vi "Main.vi"() -> ()   [LabVIEW 2017]
uses:
  Control/Virtual Damping.ctl
  88f77483-e56a-468f-9be9-12bd898d8bad.vi
  SubVI/Global.vi
panel:
  in  "beta":dbl=0.1
  in  "Survival Rate":dbl=0.5
  in  "min(Virtual Damping)":dbl=0.5
  in  "max(Virtual Damping)":dbl=3.5
  out "Fitness Value":dbl[](array[numeric])=[0.120637, 0.055035]
  out "Population":dbl[](array[numeric])=[2.8446050566710155, 2.844440959853998, 2.8444573695357, 2.844440959853998, 2.8445886469893136, 2.8446050566710155, 2.844605056671015, 2.860850641555683]
  out "Generation":i32=6
  in  "Trials per Gen.":i32=8 min=1
  out "Trial":i32=43
  in  "Trial Time (s)":dbl=10.0 format="%#_13g"
  out "Virtual Damping":T1={"bR"=4503599627370496.0, "bP"=2.8444573695357, "bY"=4503599627370496.0}
  in  "string":string="C:\\Users\\AWEAR\\Documents\\Blender"
  in  "Epsilon (deg)":dbl=2.5
  in  "Motion (deg)":dbl=75.0 format="%#_13g"
  in  "Type":enum16{"Mini45", "Joystick", "Simulation"}(ring)=enum."Joystick"
  out "error out":errorcluster
  in  "Stop":bool
  in  "error in":errorcluster
  in  "Exit":bool
  in  "Start":bool
  in  "ADL":u16(ring)=2 items=["None", "Book", "Pitcher", "Laptop", "Gear"]
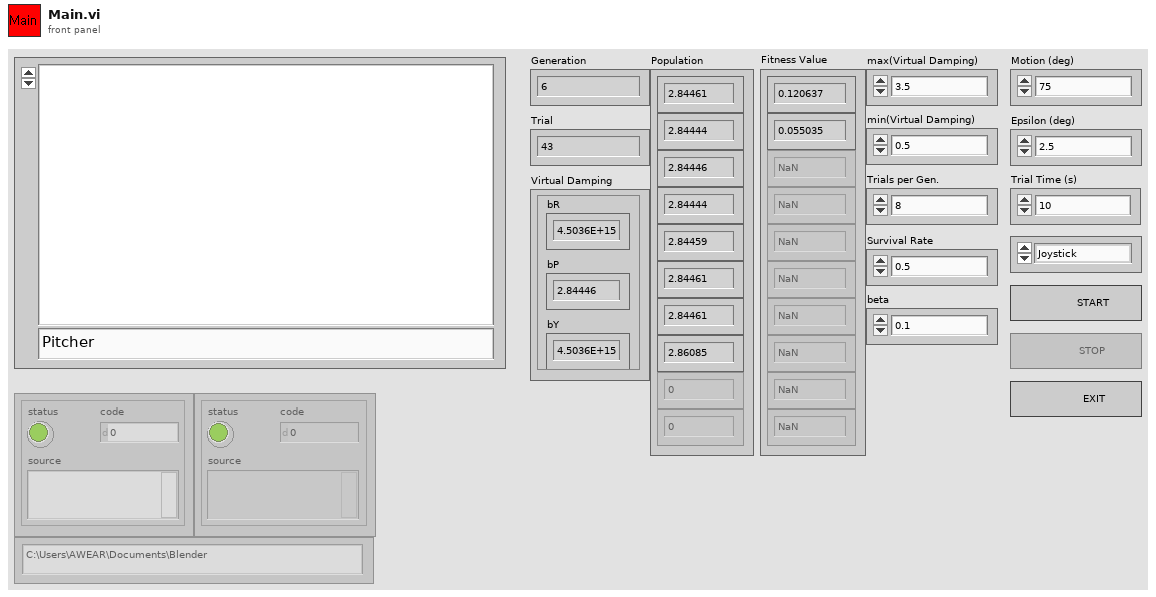
[diagram p1: front panel]
types:
  T1 = typedef "Virtual Damping.ctl" = cluster{"bR":dbl, "bP":dbl, "bY":dbl}
  T2 = enum8{"Enabled", "Disabled", "Disabled and Grayed Out"}
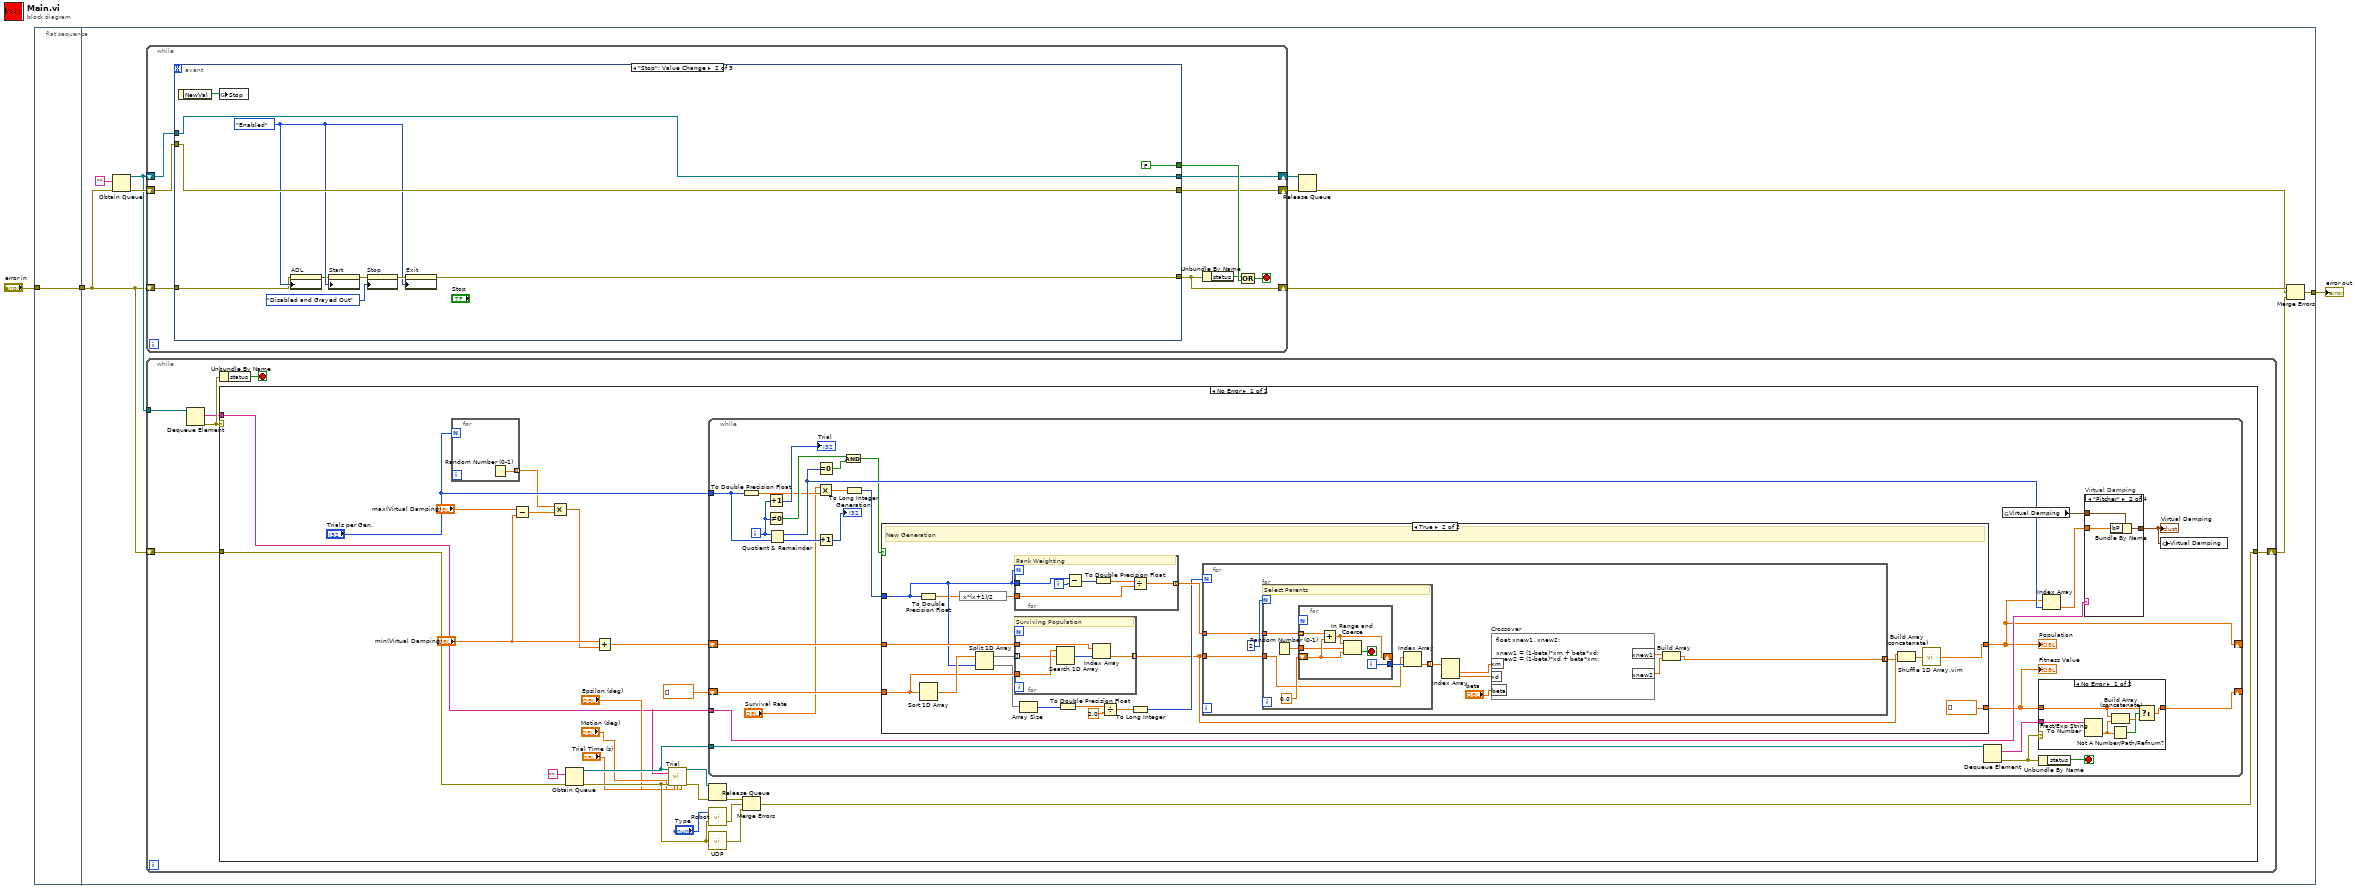
[diagram p0: block diagram]
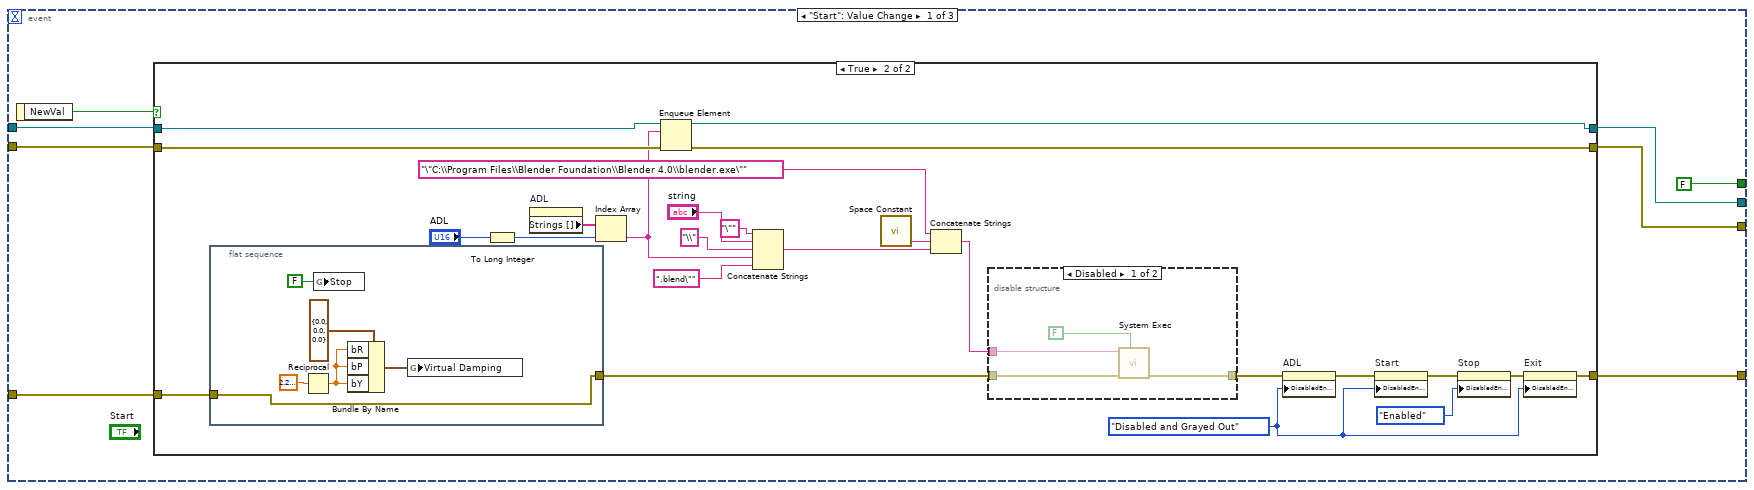
[diagram p2: hidden frame]
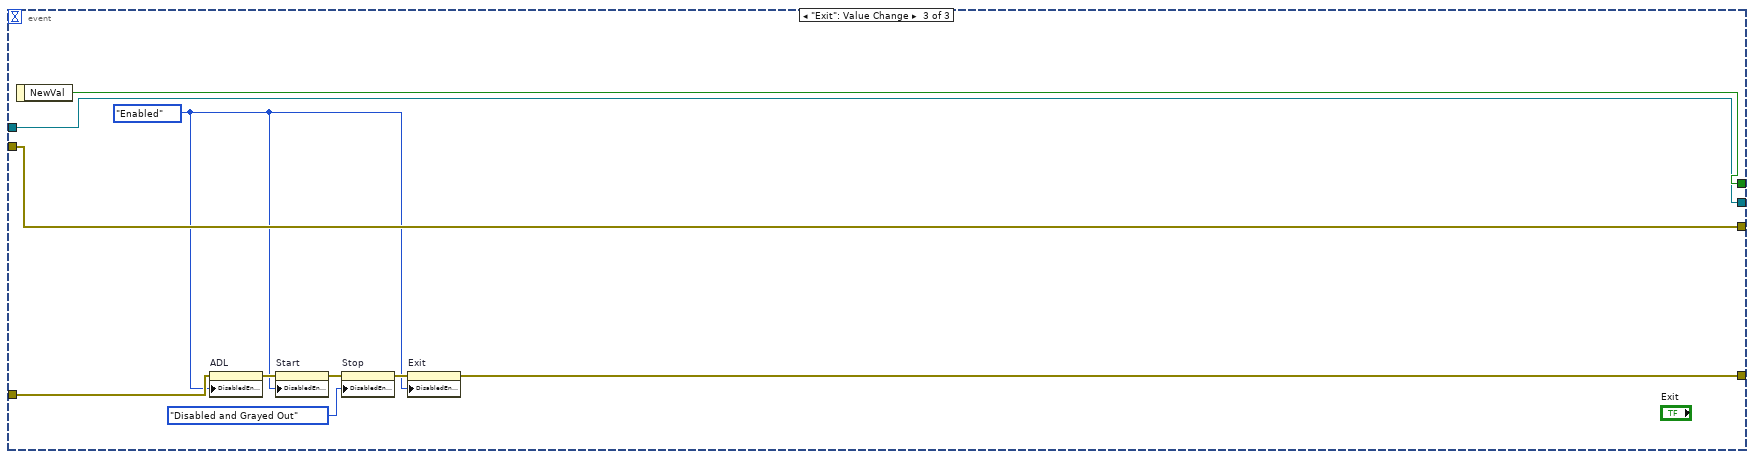
[diagram p5: hidden frame]
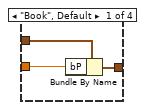
[diagram p6: hidden frame]
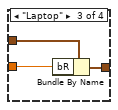
[diagram p7: hidden frame]
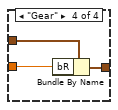
[diagram p8: hidden frame]
diagram:
  n1 = flat-sequence {
    tunnel: "error in" -> [w4]
    tunnel: [w4] -> w1
    tunnel: [w7] -> w3
    tunnel: w1 -> [w5]
    frame #0 {
    }
    frame #1 {
      n2 = Obtain Queue(element data type="", error in (no error)=w5) -> (queue out=w10:refnum<queue>, error out=w13:errorcluster)  [unwired: 3 in, 1 out]
      n3 = while {
        shift-right: [w22] -> w9
        shift-left: w5 -> [w23]
        shift-right: [w15] -> w11
        shift-left: w13 -> [w17]
        shift-right: [w16] -> w12
        shift-left: w10 -> [w18]
        stop <- w19 stop-if-true
        n4 = event shown="[1] \"Stop\": Value Change" {
          selector: _ -> [_ _ _]
          dyn-events: _ -> [_ _ _]
          timeout: _ -> [_ _ _]
          tunnel: [w30 w77 w84] -> w22
          tunnel: w23 -> [w29 w72 w88]
          tunnel: [FALSE ("Stop") FALSE ("NewVal") w91] -> w21
          tunnel: w18 -> [w27 w78 w90]
          tunnel: w17 -> [w26 w79 w89]
          tunnel: [w25 w78 w90] -> w16
          tunnel: [w24 w79 w89] -> w15
          event "Start": Value Change {
            n5 = event-data() -> ("NewVal"=w31:bool)  [unwired: 1 in]
            n6 = case shown="True" w31 {
              tunnel: [w34 w38] -> w30
              tunnel: w29 -> [w34 w50]
              tunnel: w27 -> [w32 w59]
              tunnel: w26 -> [w33 w58]
              tunnel: [w32 w57] -> w25
              tunnel: [w33 w56] -> w24
              frame False {
              }
              frame True {
                w51 = T2."Disabled and Grayed Out" ("Disabled")
                n7 = flat-sequence {
                  tunnel: [w65] -> w49
                  tunnel: w50 -> [w65]
                  frame #0 {
                    n8 = Reciprocal(x=2.220446049250313e-16) -> (1/x=w66:dbl)
                    n9 = global write "Global.vi" "Stop"(FALSE ("Stop")) -> ()
                    n10 = Bundle By Name(cluster=T1 {"bR"=0.0, "bP"=0.0, "bY"=0.0} ("Virtual Damping"), "bR"=w66, "bP"=w66, "bY"=w66) -> (w67:T1)
                    n11 = global write "Global.vi" "Virtual Damping"(w67) -> ()
                  }
                }
                n12 = To Long Integer(number="ADL") -> (32bit integer=w41:i32)
                n13 = property on="ADL" class="Ring (strict)"() -> ("Strings []"=w48:string[])  [unwired: 2 in, 2 out]
                n14 = Index Array(array=w48, index=w41) -> (element=w35:string)
                n15 = Enqueue Element(queue=w59, element=w35, error in (no error)=w58) -> (queue out=w57:refnum<queue>, error out=w56:errorcluster)  [unwired: 1 in, 1 out]
                n16 = Concatenate Strings("\"" ("string"), "string", "\\" ("string"), w35, ".blend\"" ("string")) -> (w43:string)
                n17 = call <vilib>:"Space Constant.vi"() -> ("String"=w44:string)
                n18 = Concatenate Strings("\"C:\\Program Files\\Blender Foundation\\Blender 4.0\\blender.exe\"" ("Blender Path"), w44, w43) -> (w42:string)
                n19 = disable-structure shown="Disabled" {
                  disable-tunnel: [w63 w64] -> w55
                  disable-tunnel: w49 -> [w62 w64]
                  disable-tunnel: w42 -> [w60 _]
                  frame Disabled {
                    n20 = call <vilib>:"System Exec.vi"("wait until completion? (T)"=FALSE, "error in (no error)"=w62, "command line"=w60) -> ("error out"=w63:errorcluster)  [unwired: 5 in, 3 out]
                  }
                  frame Enabled {
                  }
                }
                n21 = property on="ADL" class="Ring (strict)"(error in=w55, "DisabledEnum"=w51) -> (error out=w37:errorcluster)  [unwired: 1 in, 1 out]
                n22 = property on="Start" class="Bool"(error in=w37, "DisabledEnum"=w51) -> (error out=w54:errorcluster)  [unwired: 1 in, 1 out]
                n23 = property on="Stop" class="Bool"(error in=w54, "DisabledEnum"=T2."Enabled" ("Disabled")) -> (error out=w53:errorcluster)  [unwired: 1 in, 1 out]
                n24 = property on="Exit" class="Bool"(error in=w53, "DisabledEnum"=w51) -> (error out=w38:errorcluster)  [unwired: 1 in, 1 out]
              }
            }
          }
          event "Stop": Value Change {
            w73 = T2."Enabled" ("Disabled")
            n25 = event-data() -> ("NewVal"=w81:bool)  [unwired: 1 in]
            n26 = global write "Global.vi" "Stop"(w81) -> ()
            n27 = property on="ADL" class="Ring (strict)"(error in=w72, "DisabledEnum"=w73) -> (error out=w71:errorcluster)  [unwired: 1 in, 1 out]
            n28 = property on="Start" class="Bool"(error in=w71, "DisabledEnum"=w73) -> (error out=w76:errorcluster)  [unwired: 1 in, 1 out]
            n29 = property on="Stop" class="Bool"(error in=w76, "DisabledEnum"=T2."Disabled and Grayed Out" ("Disabled")) -> (error out=w75:errorcluster)  [unwired: 1 in, 1 out]
            n30 = property on="Exit" class="Bool"(error in=w75, "DisabledEnum"=w73) -> (error out=w77:errorcluster)  [unwired: 1 in, 1 out]
          }
          event "Exit": Value Change {
            w83 = T2."Enabled" ("Disabled")
            n31 = event-data() -> ("NewVal"=w91:bool)  [unwired: 1 in]
            n32 = property on="ADL" class="Ring (strict)"(error in=w88, "DisabledEnum"=w83) -> (error out=w85:errorcluster)  [unwired: 1 in, 1 out]
            n33 = property on="Start" class="Bool"(error in=w85, "DisabledEnum"=w83) -> (error out=w87:errorcluster)  [unwired: 1 in, 1 out]
            n34 = property on="Stop" class="Bool"(error in=w87, "DisabledEnum"=T2."Disabled and Grayed Out" ("Disabled")) -> (error out=w86:errorcluster)  [unwired: 1 in, 1 out]
            n35 = property on="Exit" class="Bool"(error in=w86, "DisabledEnum"=w83) -> (error out=w84:errorcluster)  [unwired: 1 in, 1 out]
          }
        }
        n36 = Unbundle By Name(w22) -> ("status"=w20:bool)
        n37 = Compound Arithmetic op=OR(w20, w21) -> (w19:bool)
      }
      n38 = while {
        tunnel: w10 -> [w97]
        shift-right: [w94] -> w6
        shift-left: w5 -> [w93]
        stop <- w95 stop-if-true
        n39 = Dequeue Element(queue=w97) -> (element=w92:string, error out=w96:errorcluster)  [unwired: 2 in, 2 out]
        n40 = Unbundle By Name(w96) -> ("status"=w95:bool)
        n41 = case shown="No Error" w96 {
          tunnel: [w119 w221] -> w94
          tunnel: w93 -> [w118 w221]
          tunnel: w92 -> [w106 _]
          frame No Error {
            n42 = for {
              N: "Trials per Gen." -> [_]
              tunnel: [w121] -> w101 mode=indexing
              n43 = Random Number (0-1)() -> (number: 0 to 1=w121:dbl)
            }
            n44 = Subtract(x="max(Virtual Damping)", y="min(Virtual Damping)") -> (x-y=w100:dbl)
            n45 = Multiply(x=w101, y=w100) -> (x*y=w99:dbl[])
            n46 = Obtain Queue(element data type="", error in (no error)=w118) -> (queue out=w113:refnum<queue>, error out=w111:errorcluster)  [unwired: 3 in, 1 out]
            n47 = Add(x="min(Virtual Damping)", y=w99) -> (x+y=w98:dbl[])
            n48 = call "Trial.vi"("queue in"=w113, "ADL"=w106, "error in (no error)"=w111, "Motion (deg)"="Motion (deg)", "Epsilon (deg)"="Epsilon (deg)", "Trial Time (s)"="Trial Time (s)") -> ("queue out"=w112:refnum<queue>, "error out"=w108:errorcluster)  [unwired: 8 in]
            n49 = while {
              tunnel: w113 -> [w146]
              tunnel: "Trials per Gen." -> [w126]
              shift-right: [w136] -> _
              shift-left: w98 -> [w141]
              tunnel: w106 -> [w139]
              shift-right: [w128] -> _
              shift-left: dbl[] [] -> [w129]
              i -> [w133]
              stop <- w145 stop-if-true
              n50 = To Double Precision Float(number=w126) -> (double precision float=w125:dbl)
              n51 = Increment(x=w133) -> (x+1=→"Trial":i32)
              n52 = Not Equal To 0?(x=w133) -> (x != 0?=w131:bool)
              n53 = Quotient & Remainder(x=w133, y=w126) -> (x-y*floor(x/y)=w140:i32, floor(x/y)=w143:i32)
              n54 = Multiply(x="Survival Rate", y=w125) -> (x*y=w123:dbl)
              n55 = Equal To 0?(x=w140) -> (x = 0?=w132:bool)
              n56 = Increment(x=w143) -> (x+1=→"Generation":i32)
              n57 = And(x=w131, y=w132) -> (x .and. y?=w130:bool)
              n58 = To Long Integer(number=w123) -> (32bit integer=w122:i32)
              n59 = case shown="True" w130 {
                tunnel: w141 -> [w161 w177]
                tunnel: [w161 w162] -> w136
                tunnel: w129 -> [w160 w179]
                tunnel: [w160 dbl[] []] -> w127
                tunnel: w122 -> [_ w176]
                frame False {
                }
                frame True {
                  # "New Generation"
                  n60 = To Double Precision Float(number=w176) -> (double precision float=w175:dbl)
                  n61 = Sort 1D Array(array=w179) -> (sorted array=w180:dbl[])
                  n62 = expression code="x*(x+1)/2"(w175) -> (w174:dbl)
                  n63 = Split 1D Array(array=w180, index=w176) -> (first subarray=w178:dbl[], second subarray=w172:dbl[])
                  n64 = for {
                    N: w176 -> [_]
                    tunnel: w176 -> [w208]
                    tunnel: w174 -> [w204]
                    tunnel: [w203] -> w173 mode=indexing
                    i -> [w207]
                    # "Rank Weighting"
                    n65 = Subtract(x=w208, y=w207) -> (x-y=w206:i32)
                    n66 = To Double Precision Float(number=w206) -> (double precision float=w205:dbl)
                    n67 = Divide(x=w205, y=w204) -> (x/y=w203:dbl)
                  }
                  n68 = for {
                    tunnel: w179 -> [w213]
                    tunnel: w178 -> [w212] mode=indexing
                    tunnel: w177 -> [w210]
                    tunnel: [w209] -> w165 mode=indexing
                    # "Surviving Population"
                    n69 = Search 1D Array(1D array=w213, element=w212) -> (index of element=w211:i32)  [unwired: 1 in]
                    n70 = Index Array(array=w210, index=w211) -> (element=w209:dbl)
                  }
                  n71 = Array Size(array=w172) -> (size(s)=w171:i32)
                  n72 = To Double Precision Float(number=w171) -> (double precision float=w170:dbl)
                  n73 = Divide(x=w170, y=2.0) -> (x/y=w168:dbl)
                  n74 = To Long Integer(number=w168) -> (32bit integer=w167:i32)
                  n75 = for {
                    N: w167 -> [_]
                    tunnel: w173 -> [w189]
                    tunnel: w165 -> [w188]
                    tunnel: [w181] -> w164 mode=concatenating
                    n76 = for {
                      N: 2 -> [_]
                      tunnel: w189 -> [w196]
                      tunnel: w188 -> [w192]
                      tunnel: [w191] -> w187 mode=indexing
                      # "Select Parents"
                      n77 = Random Number (0-1)() -> (number: 0 to 1=w195:dbl)
                      n78 = for {
                        tunnel: w196 -> [w202] mode=indexing
                        tunnel: w195 -> [w199]
                        shift-right: [w200] -> _
                        shift-left: 0.0 -> [w201]
                        tunnel: [w197] -> w193
                        i -> [w197]
                        stop <- w198 stop-if-true
                        n79 = Add(x=w202, y=w201) -> (x+y=w200:dbl)
                        n80 = In Range and Coerce(upper limit=w200, x=w199, lower limit=w201) -> (In Range?=w198:bool)  [unwired: 1 out]
                      }
                      n81 = Index Array(array=w192, index=w193) -> (element=w191:dbl)
                    }
                    n82 = Index Array(array=w187) -> (element #1=w185:dbl, element #2=w184:dbl)  [unwired: 2 in]
                    n83 = formula code="float xnew1, xnew2;\n\nxnew1 = (1-beta)*xm + beta*xd;\nxnew2 = (1-beta)*xd + beta*xm;" "Crossover"("xm"=w185, "xd"=w184, "beta"="beta") -> ("xnew1"=w183:dbl, "xnew2"=w182:dbl)
                    n84 = Build Array(w183, w182) -> (w181:dbl[])
                  }
                  n85 = Build Array (concatenate)(w165, w164) -> (w163:dbl[])
                  n86 = call "Shuffle 1D Array.vim"("array"=w163) -> ("shuffled array"=w162:dbl[])  [unwired: 4 in]
                }
              }
              "Population" <- w136
              "Fitness Value" <- w127
              n87 = Dequeue Element(queue=w146) -> (element=w134:string, error out=w147:errorcluster)  [unwired: 2 in, 2 out]
              n88 = global read "Global.vi" "Virtual Damping"() -> (w135:T1)
              n89 = case shown="No Error" w147 {
                tunnel: w134 -> [w219 _]
                tunnel: [w216 w220] -> w128
                tunnel: w127 -> [w215 w220]
                frame No Error {
                  n90 = Fract/Exp String To Number(string=w219) -> (number=w218:dbl)  [unwired: 3 in, 1 out]
                  n91 = Not A Number/Path/Refnum?(number/path/refnum=w218) -> (NaN/Path/Refnum?=w217:bool)
                  n92 = Build Array (concatenate)(w215, w218) -> (w214:dbl[])
                  n93 = Select(t=w215, s=w217, f=w214) -> (s? t:f=w216:dbl[])
                }
                frame Error {
                }
              }
              n94 = Unbundle By Name(w147) -> ("status"=w145:bool)
              n95 = Index Array(array=w136, index=w140) -> (element=w138:dbl)
              n96 = case "Virtual Damping" shown="\"Pitcher\"" w139 {
                tunnel: w135 -> [w150 w153 w156 w159]
                tunnel: w138 -> [w149 w152 w155 w158]
                tunnel: [w148 w151 w154 w157] -> w137
                frame "Book", Default {
                  n97 = Bundle By Name(cluster=w150, "bP"=w149) -> (w148:T1)
                }
                frame "Pitcher" {
                  n98 = Bundle By Name(cluster=w153, "bP"=w152) -> (w151:T1)
                }
                frame "Laptop" {
                  n99 = Bundle By Name(cluster=w156, "bR"=w155) -> (w154:T1)
                }
                frame "Gear" {
                  n100 = Bundle By Name(cluster=w159, "bR"=w158) -> (w157:T1)
                }
              }
              "Virtual Damping" <- w137
              n101 = global write "Global.vi" "Virtual Damping"(w137) -> ()
            }
            n102 = Release Queue(queue=w112, error in (no error)=w108) -> (error out=w116:errorcluster)  [unwired: 1 in, 2 out]
            n103 = call "Robot.vi"("error in"=w111, "Type"="Type") -> ("error out"=w115:errorcluster)  [unwired: 1 in]
            n104 = call "UDP.vi"("error in (no error)"=w111) -> ("error out"=w120:errorcluster)
            n105 = Merge Errors(w116, w115, w120) -> (w119:errorcluster)
          }
          frame Error {
          }
        }
      }
      n106 = Release Queue(queue=w12, error in (no error)=w11) -> (error out=w8:errorcluster)  [unwired: 1 in, 2 out]
      n107 = Merge Errors(w9, w8, w6) -> (w7:errorcluster)
    }
  }
  "error out" <- w3
